vi "GetDefaultParams.vi"(8 "error in (no error)":errorcluster, 10 "Path":path, 11 "MultiBandState in":refnum<class "MultiBandState.lvclass">) -> (0 "error out":errorcluster, 3 "MultiBandState out":refnum<class "MultiBandState.lvclass">)   [LabVIEW 2014, in "Functions.lvlib" / "MultiBandState.lvclass"]
uses:
  MultiBandState.lvclass
  TypeDefs/clMultiBandConfig.ctl
  TypeDefs/MultiBandConfig.ctl
  FunctionBaseClass/FunctionBase.lvclass/FunctionBase.ctl
  MultiBandState.lvclass/MultiBandState.ctl
  FunctionBaseClass/Accessors/Read FunctionIniFilePath.vi
  Accessors/Write MultiBandConfig.vi
  FunctionBaseClass/FunctionBase.lvclass
  <vilib>/Utility/config.llb/NI_LVConfig.lvlib
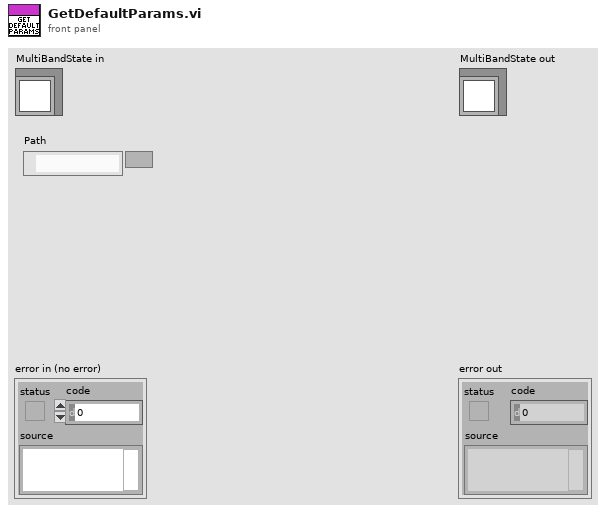
[diagram p1: front panel]
types:
  T1 = typedef "Functions.lvlib/MultiBandState.lvclass/clMultiBandConfig.ctl" = cluster{"Count":i32, "MultiBandConfig":T2[]}
  T2 = typedef "Functions.lvlib/MultiBandState.lvclass/MultiBandConfig.ctl" = cluster{"Handle":string, "Type":enum16{"Multiband", "Amplitude Modulation", "Phase Modulation", "Combined Modulation"}, "Freq":dbl[], "Index":dbl[], "Phase":dbl[][], "Damping":dbl[]}
  T3 = typedef "NI_LVConfig.lvlib/Config Data RefNum.ctl" = refnum<k1>
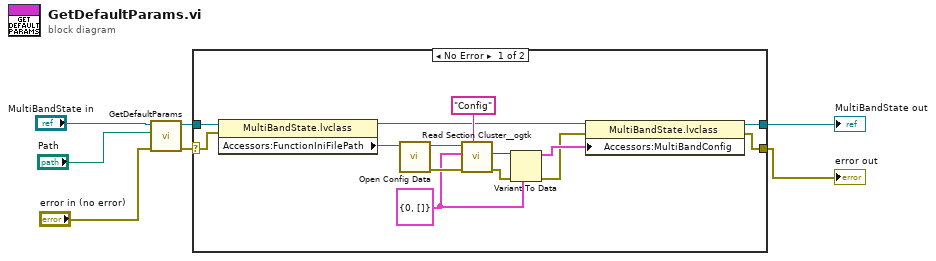
[diagram p0: block diagram]
diagram:
  n1 = call-parent "GetDefaultParams.vi"("error in (no error)"="error in (no error)", "Path"="Path", "FunctionBase in"="MultiBandState in") -> ("error out"=w4:errorcluster, "FunctionBase out"=w3:refnum<class "MultiBandState.lvclass">)  [unwired: 7 in]
  n2 = case shown="No Error" w4 {
    selector: w4 -> [w21 w22]
    tunnel: [w12 w23] -> w2
    tunnel: w3 -> [w20 w23]
    tunnel: [w8 w22] -> w1
    frame No Error {
      w13 = T1 {"Count"=0, "MultiBandConfig"=[]} ("clMultiBandConfig")
      n3 = property class="MultiBandState.lvclass"(reference=w20, error in=w21) -> (reference out=w9:refnum<class "MultiBandState.lvclass">, "Accessors:FunctionIniFilePath"=w19:path)  [unwired: 1 out]
      n4 = call <vilib>:"Open Config Data.vi"("configuration file path"=w19) -> ("error out"=w18:errorcluster, "refnum"=w17:T3)  [unwired: 8 in, 1 out]
      n5 = call <userlib>:"Read Section Cluster__ogtk.vi"("section (optional)"="Config", "error in (no error)"=w18, "Section Formatted Cluster Type"=w13, "refnum"=w17) -> ("error out"=w15:errorcluster, "Section Formatted Cluster"=w14:variant)  [unwired: 3 in, 3 out]
      n6 = Variant To Data(error in=w15, type=w13, Variant=w14) -> (data=w11:T1, error out=w10:errorcluster)
      n7 = property class="MultiBandState.lvclass"(reference=w9, error in=w10, "Accessors:MultiBandConfig"=w11) -> (reference out=w12:refnum<class "MultiBandState.lvclass">, error out=w8:errorcluster)
    }
    frame Error {
    }
  }
  "error out" <- w1
  "MultiBandState out" <- w2
